vi "byebyeMethod.vi"(1 "device description":T1) -> ()   [LabVIEW 2010]
uses:
  <vilib>/Utility/tcp.llb/UDP Multicast Write-Only Open.vi
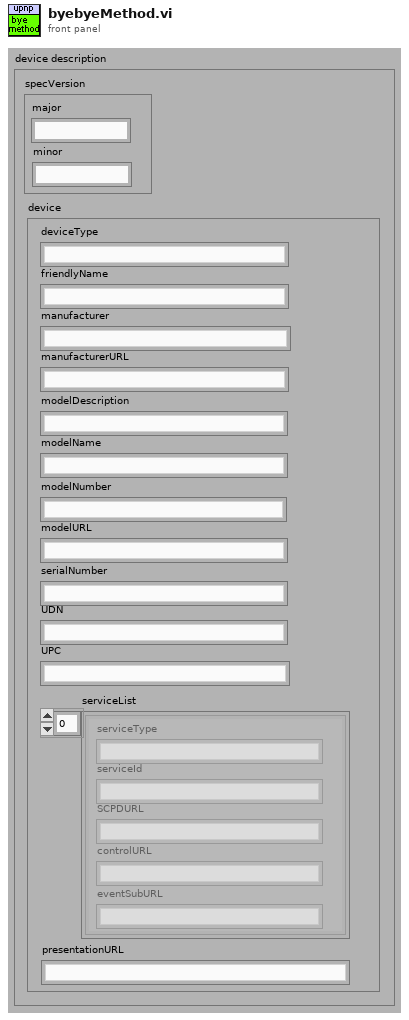
[diagram p1: front panel]
types:
  T1 = cluster{"specVersion":cluster{"major":string, "minor":string}, "device":cluster{"deviceType":string, "friendlyName":string, "manufacturer":string, "manufacturerURL":string, "modelDescription":string, "modelName":string, "modelNumber":string, "modelURL":string, "serialNumber":string, "UDN":string, "UPC":string, "serviceList":cluster{"serviceType":string, "serviceId":string, "SCPDURL":string, "controlURL":string, "eventSubURL":string}[], "presentationURL":string}}
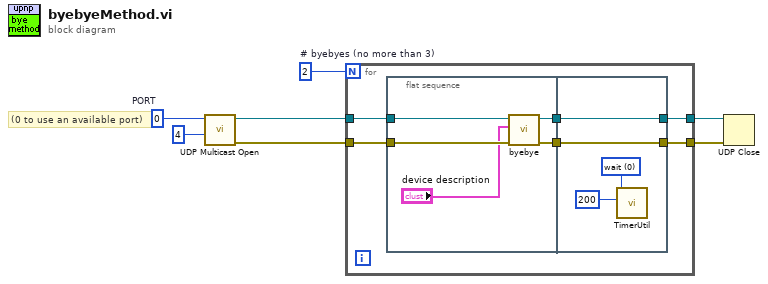
[diagram p0: block diagram]
diagram:
  w1 = 2  # # byebyes (no more than 3)
  w7 = u16 0  # PORT
  # "(0 to use an available port)"
  n1 = call-poly <vilib>:"UDP Multicast Open.vi"("time-to-live (1)"=u16 4, "port"=w7) -> ("error out"=w4:errorcluster, "connection ID"=w3:refnum<k16>)  [unwired: 2 in, 6 out]
  n2 = for {
    N: w1 -> [_]
    tunnel: w3 -> [w13]
    tunnel: w4 -> [w12]
    tunnel: [w10] -> w5
    tunnel: [w8] -> w6
    n3 = flat-sequence {
      tunnel: w13 -> [w18]
      tunnel: w12 -> [w15]
      tunnel: [w17] -> w11
      tunnel: [w16] -> w9
      tunnel: [w20] -> w10
      tunnel: w11 -> [w20]
      tunnel: [w19] -> w8
      tunnel: w9 -> [w19]
      frame #0 {
        n4 = call "byebye.vi"("error in (no error)"=w15, "root"="device description", "connection ID"=w18) -> ("error out"=w16:errorcluster, "connection ID out"=w17:refnum<k16>)  [unwired: 7 out]
      }
      frame #1 {
        w22 = u16 0 items=["wait", "waitRandom"] ("typeTimer")
        n5 = call "TimerUtil.vi"("time (msec)"=u32 200, "typeTimer"=w22) -> ()  [unwired: 10 out]
      }
    }
  }
  n6 = UDP Close(connection ID=w5, 8:w6) -> ()  [unwired: 2 out]
